vi "VeriStand Framework Configuration.Create.vi"(8 "error in (no error)":errorcluster, 10 "configuration path":path, 11 "Device Item Ref":T1=18446744073709551615 format="%.0x") -> (0 "error out":errorcluster, 3 "VeriStand Framework Configuration":refnum<class "VeriStand DSF.Framework.Configuration.lvclass">)   [LabVIEW 2017, in "Data Sharing Custom Device Engine.lvlib" / "VeriStand DSF.Framework.Configuration.lvclass"]
uses:
  VeriStand DSF.Framework.Configuration.lvclass
  <vilib>/NI Veristand/Custom Device API/Custom Device Item Ref.ctl
  VeriStand DSF.Framework.Configuration.lvclass/VeriStand DSF.Framework.Configuration.ctl
  VeriStand DSF.Plugin.Configuration.lvclass
  C:/Builds/Data Sharing Framework/Current/Data Sharing Framework Core/DSF Core.lvlibp/Shared/Classes/Plugin/Plugin Configuration.lvclass
  <vilib>/NI Veristand/Custom Device API/Custom Device API.lvlib
  VeriStand DSF.Transfer Group.Configuration.lvclass
  VeriStand DSF.Transfer.Configuration.lvclass
  Builds/Data Sharing Framework/Current/Data Sharing Framework Core/DSF Core.lvlibp/Shared/Classes/Framework/Framework Configuration.lvclass
  C:/Builds/Data Sharing Framework/Current/Data Sharing Framework Core/DSF Core.lvlibp/Shared/Classes/Framework/Framework Configuration.lvclass
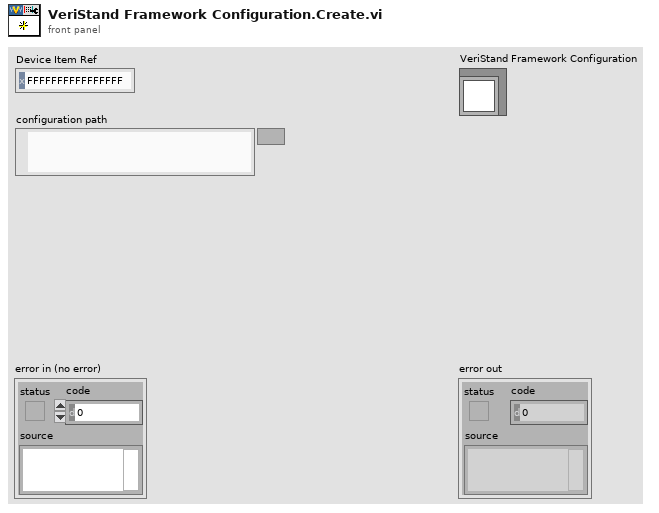
[diagram p1: front panel]
types:
  T1 = typedef "Custom Device API.lvlib/Custom Device Item Ref.ctl" = u64
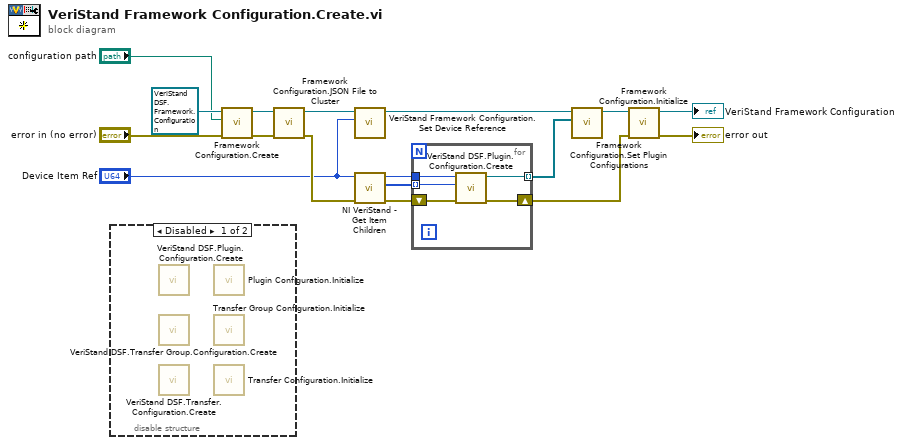
[diagram p0: block diagram]
diagram:
  n1 = disable-structure shown="Disabled" {
    frame Disabled {
      n2 = call "VeriStand DSF.Plugin.Configuration.Create.vi"() -> ()  [unwired: 10 in, 2 out]
      n3 = call "VeriStand DSF.Transfer Group.Configuration.Create.vi"() -> ()  [unwired: 10 in, 2 out]
      n4 = call "VeriStand DSF.Transfer.Configuration.Create.vi"() -> ()  [unwired: 10 in, 2 out]
      n5 = call-dynamic "Plugin Configuration.Initialize.vi"() -> ()  [unwired: 10 in, 2 out]
      n6 = call-dynamic "Transfer Group Configuration.Initialize.vi"() -> ()  [unwired: 10 in, 2 out]
      n7 = call-dynamic "Transfer Configuration.Initialize.vi"() -> ()  [unwired: 10 in, 2 out]
    }
    frame Enabled {
    }
  }
  n8 = call "Framework Configuration.Create.vi"("error in (no error)"="error in (no error)", "configuration path"="configuration path", "Framework Configuration type"=refnum<class "VeriStand DSF.Framework.Configuration.lvclass"> refnum ("VeriStand Framework Configuration")) -> ("error out"=w9:errorcluster, "Framework Configuration"=w15:refnum<class "VeriStand DSF.Framework.Configuration.lvclass">)  [unwired: 7 in]
  n9 = call "Framework Configuration.JSON File to Cluster.vi"("error in (no error)"=w9, "Framework Configuration in"=w15) -> ("error out"=w6:errorcluster, "Framework Configuration out"=w8:refnum<class "VeriStand DSF.Framework.Configuration.lvclass">)  [unwired: 8 in]
  n10 = call "VeriStand Framework Configuration.Set Device Reference.vi"("Device Item Ref"="Device Item Ref", "VeriStand Framework Configuration in"=w8) -> ("VeriStand Framework Configuration out"=w10:refnum<class "VeriStand DSF.Framework.Configuration.lvclass">)  [unwired: 9 in]
  n11 = call <vilib>:"NI VeriStand - Get Item Children.vi"("error in (no error)"=w6, "Item Ref in"="Device Item Ref") -> ("error out"=w17:errorcluster, "Child Refs"=w5:T1[], "Item Ref out"=w3:T1)  [unwired: 6 in, 1 out]
  n12 = for {
    shift-right: [w21] -> w12
    shift-left: w17 -> [w22]
    tunnel: [w20] -> w16 mode=indexing
    tunnel: w5 -> [w19] mode=indexing
    tunnel: w3 -> [w18]
    n13 = call "VeriStand DSF.Plugin.Configuration.Create.vi"("error in (no error)"=w22, "Section Ref"=w19, "Device Ref"=w18) -> ("error out"=w21:errorcluster, "Plugin Configuration"=w20:refnum<class "VeriStand DSF.Plugin.Configuration.lvclass">)  [unwired: 7 in]
  }
  n14 = call "Framework Configuration.Set Plugin Configurations.vi"("Plugin Configurations"=w16, "Framework Configuration in"=w10) -> ("Framework Configuration out"=w14:refnum<class "VeriStand DSF.Framework.Configuration.lvclass">)  [unwired: 9 in]
  n15 = call-dynamic "Framework Configuration.Initialize.vi"("error in (no error)"=w12, "Framework Configuration in"=w14) -> ("error out"=→"error out":errorcluster, "Framework Configuration out"=→"VeriStand Framework Configuration":refnum<class "VeriStand DSF.Framework.Configuration.lvclass">)  [unwired: 8 in]
